vi "Main.vi"(11 "Module Admin":refnum<class "Delacor_lib_QMH_Module Admin.lvclass">) -> ()   [LabVIEW 2023, in "Initial Data.lvlib"]
doc: "This template is based off of the Queued Message Handler design pattern and the Queued Message Handler project template that ships with LabVIEW.\n\nThe main difference is that the queue is private to this module and communication between modules is performed via Broadcast and Request events.\n\nRequest events are wrapped in public API methods and are handled in the Event Handling Loop (EHL) of this VI. Any module can register for Broadcast events sent by this module. The EHL generates messages based on user interface actions.\n\nThe Message Handling Loop (MHL) processes messages generated by the EHL, or by other messages. The messages are string values, so new messages can be added easily to the Message Cases case structure in the MHL. Each message cluster can also provide an optional value for Message Data, which is a variant that can be converted to whatever message-specific data is required.\n_____\nBased on DQMH Project Template 6.1.0.94."
uses:
  Initial Data.lvlib
  <vilib>/Delacor/Delacor QMH/Libraries/Module Admin_class/Delacor_lib_QMH_Module Admin.lvclass
  InitalData Type.ctl
  Module Data--cluster.ctl
  <vilib>/Delacor/Delacor QMH/Libraries/Message Queue_class/Delacor_lib_QMH_Message Queue.lvclass/Delacor_lib_QMH_Message Queue.ctl
  Stop Argument--cluster.ctl
  <vilib>/Delacor/Delacor QMH/Libraries/Module Admin_class/Delacor_lib_QMH_Module Admin.lvclass/Delacor_lib_QMH_Module Admin.ctl
  Update Brod Argument--cluster.ctl
  SubPanel Argument--cluster.ctl
  <vilib>/Utility/miscctls.llb/LVPointTypeDef.ctl
  <vilib>/Delacor/Delacor QMH/Libraries/Message Queue_class/Delacor_lib_QMH_Enqueue Message (Single).vi
  <vilib>/Delacor/Delacor QMH/Libraries/Module Admin_class/Delacor_lib_QMH_Get External Launch.vi
  <vilib>/Utility/error.llb/Error Cluster From Error Code.vi
  <vilib>/ErrorRing/Error Ring.xnode
  <vilib>/Delacor/Delacor QMH/Libraries/Message Queue_class/Delacor_lib_QMH_Message Queue.lvclass
panel:
  in  "Исходные данные":T1
  out "error out":errorcluster
  in  "Simulate MHL Error":bool
  in  "Simulate EHL Error":bool
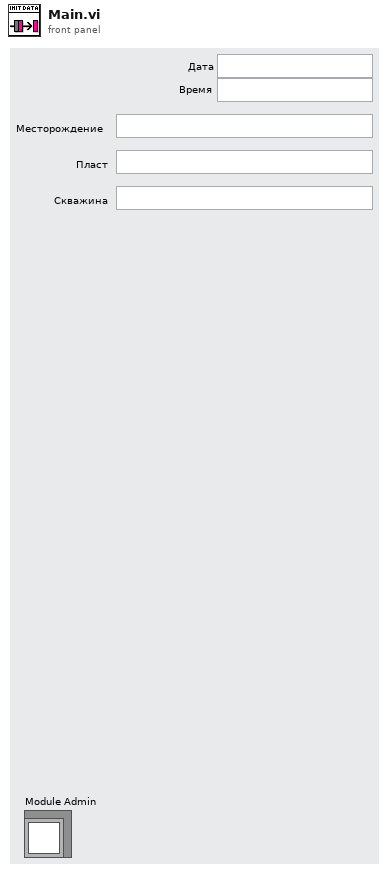
[diagram p1: front panel]
types:
  T1 = typedef "Initial Data.lvlib/InitalData Type.ctl" = cluster{"Дата":string, "Время":string, "Месторождение":string, "Пласт":string, "Скважина":string}
  T2 = typedef "Initial Data.lvlib/Request Events--cluster.ctl" = cluster{"Stop Module":refnum<user-event>, "Show Panel":refnum<user-event>, "Hide Panel":refnum<user-event>, "Get Module Execution Status":refnum<user-event>, "Show Diagram":refnum<user-event>, "Update Brod":refnum<user-event>, "SubPanel":refnum<user-event>}
  T3 = typedef "Initial Data.lvlib/Module Data--cluster.ctl" = cluster{"Status":string, "Исходные данные":T1}
  T4 = enum32{"invalid lock state", "Not Locked", "Locked (No Password)", "Password-protected"}
  T5 = typedef "Initial Data.lvlib/Stop Argument--cluster.ctl" = cluster{"Origin":string, "Exit via Stop Module Req?":bool, "Wait for Module to stop?":bool}
  T6 = typedef "Initial Data.lvlib/Update Brod Argument--cluster.ctl" = cluster{"Boolean":bool}
  T7 = typedef "Initial Data.lvlib/SubPanel Argument--cluster.ctl" = cluster{"Sub Panel":refnum<vi>}
  T8 = typedef "LVPointTypeDef.ctl" = cluster{"Horizontal":i16, "Vertical":i16}
  T9 = enum32{"Invalid", "Standard", "Closed", "Hidden", "Minimized", "Maximized"}
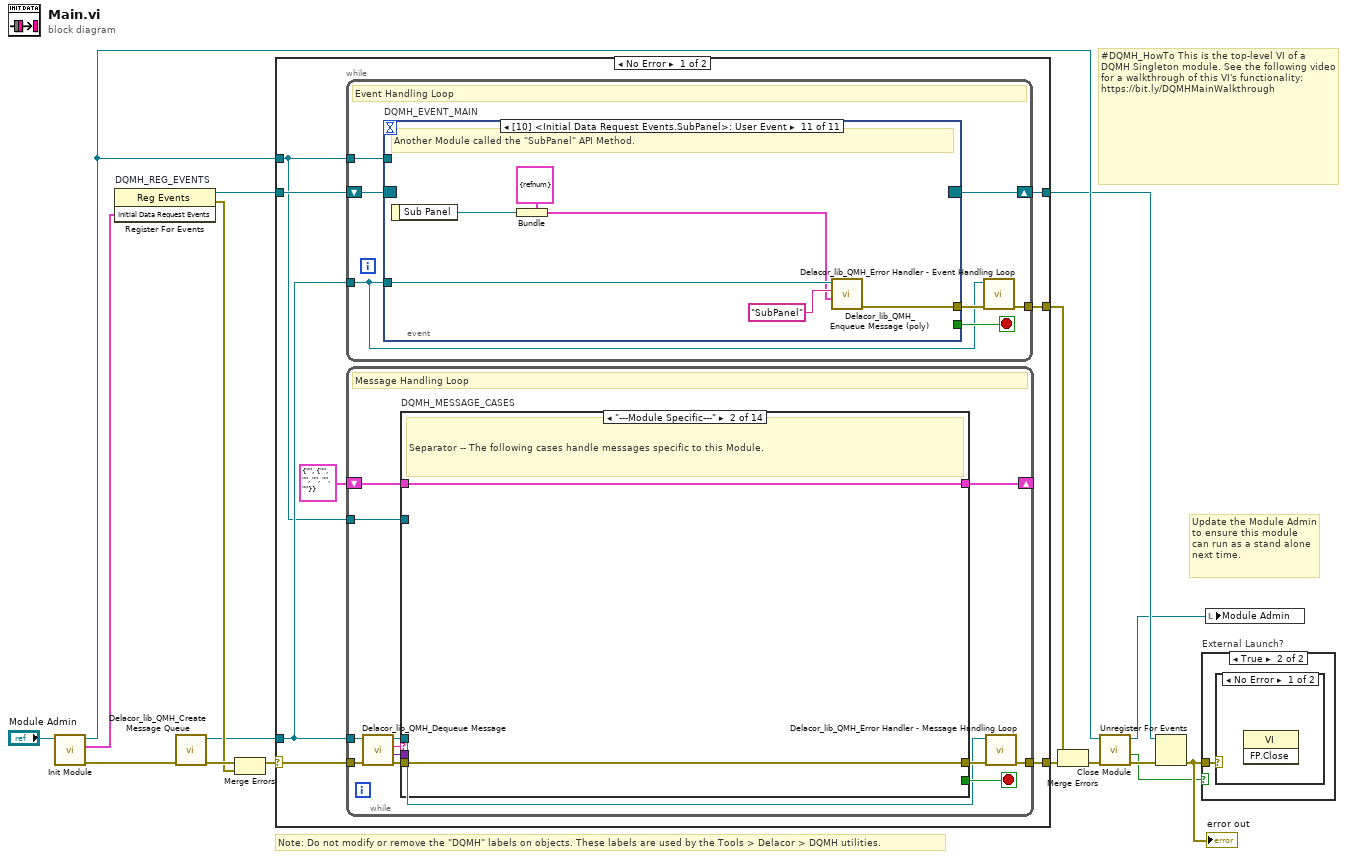
[diagram p0: block diagram]
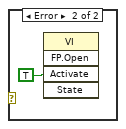
[diagram p3: hidden frame]
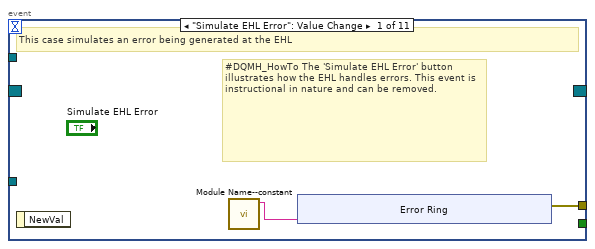
[diagram p4: hidden frame]
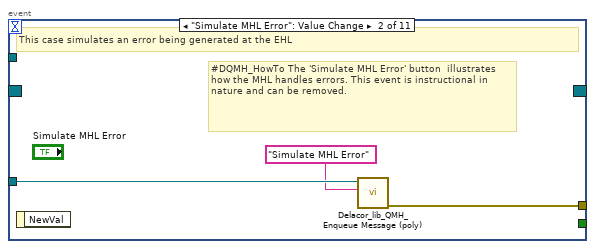
[diagram p5: hidden frame]
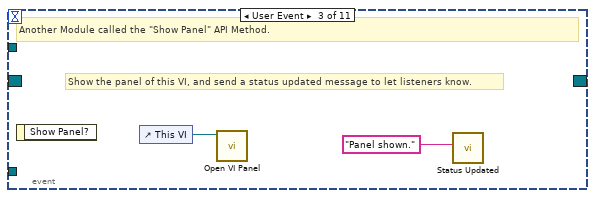
[diagram p6: hidden frame]
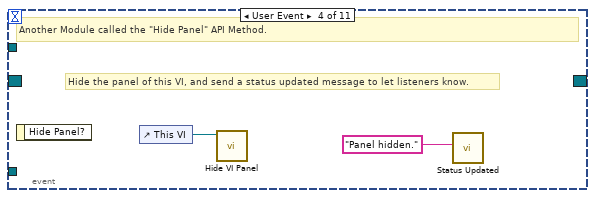
[diagram p7: hidden frame]
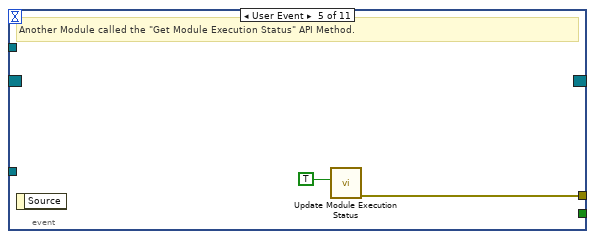
[diagram p8: hidden frame]
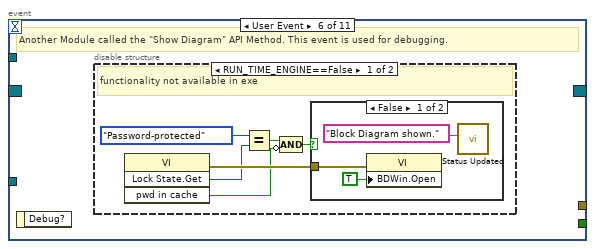
[diagram p9: hidden frame]
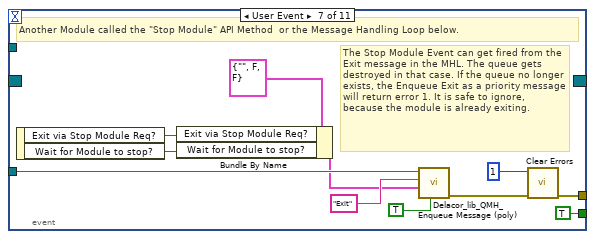
[diagram p12: hidden frame]
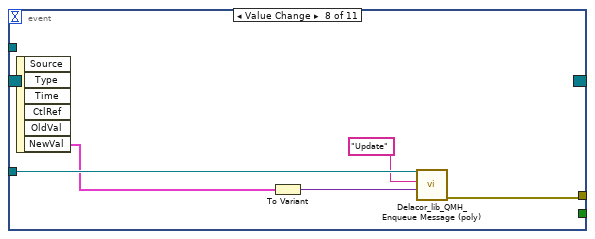
[diagram p13: hidden frame]
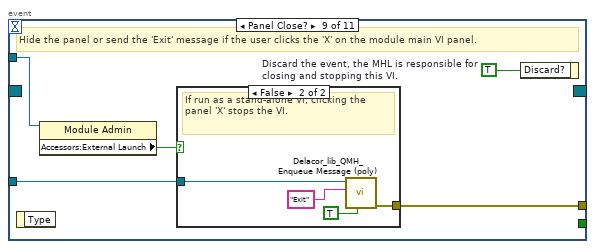
[diagram p14: hidden frame]
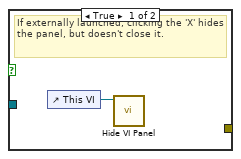
[diagram p15: hidden frame]
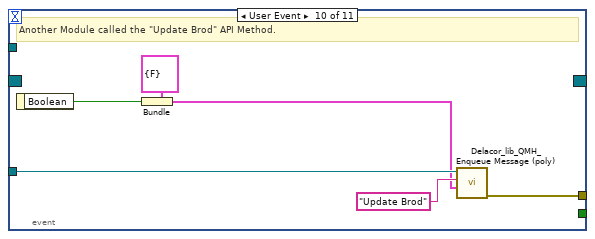
[diagram p16: hidden frame]
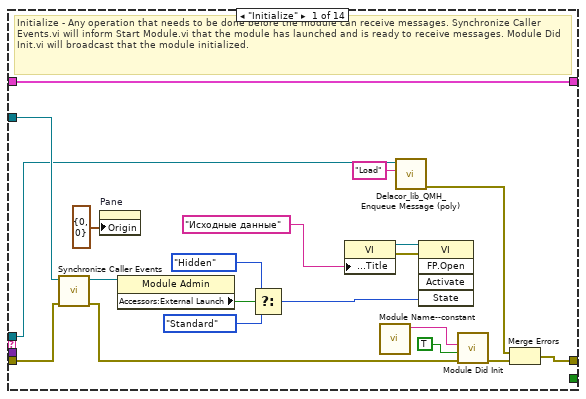
[diagram p17: hidden frame]
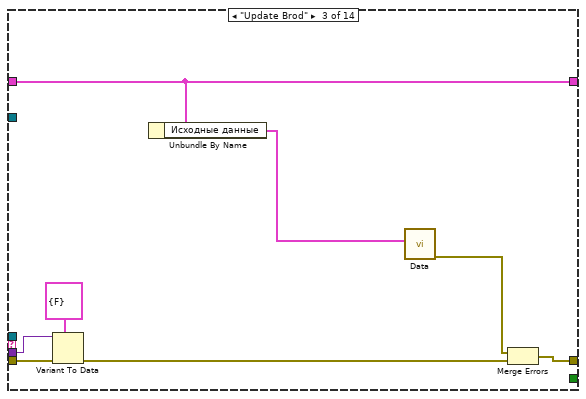
[diagram p18: hidden frame]
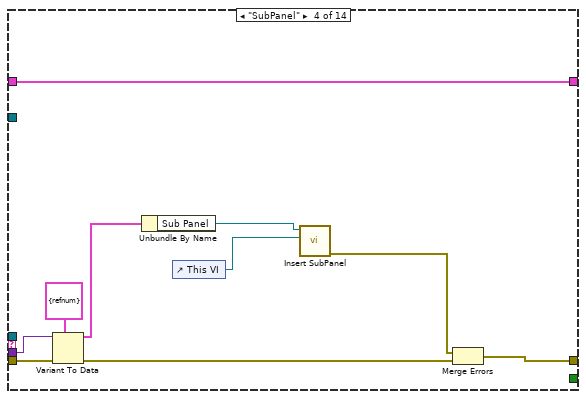
[diagram p19: hidden frame]
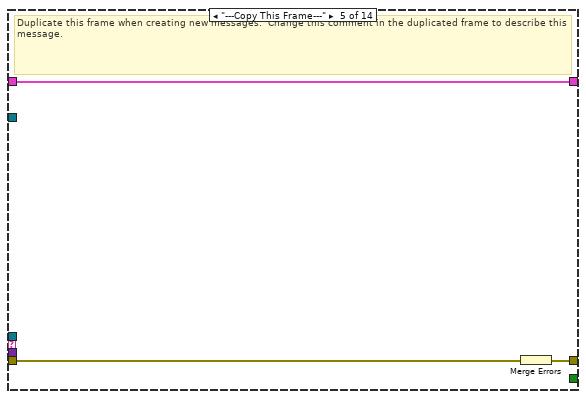
[diagram p20: hidden frame]
diagram:
  # "#DQMH_HowTo This is the top-level VI of a DQMH Singleton module. See the following video for a walkthrough of this VI's functionality: https://bit.ly/DQMHMainWalkthrough"
  # "Note: Do not modify or remove the \"DQMH\" labels on objects. These labels are used by the Tools > Delacor > DQMH utilities."
  # "Update the Module Admin to ensure this module can run as a stand alone next time."
  n1 = call "Init Module.vi"("Singleton Module Admin in"="Module Admin") -> ("error out"=w16:errorcluster, "Initial Data Request Events"=w5:T2, "Singleton Module Admin out"=w8:refnum<class "Delacor_lib_QMH_Module Admin.lvclass">)  [unwired: 8 in]
  n2 = register-events "DQMH_REG_EVENTS"(w5) -> (reference out=w6:refnum<event-registration>, error out=w9:errorcluster)  [unwired: 2 in]
  n3 = call <vilib>:"Delacor_lib_QMH_Create Message Queue.vi"("error in"=w16) -> ("error out"=w11:errorcluster, "Message Queue"=w4:refnum<class "Delacor_lib_QMH_Message Queue.lvclass">)  [unwired: 9 in]
  n4 = Merge Errors(w11, w9) -> (w10:errorcluster)
  n5 = case shown="No Error" w10 {
    selector: w10 -> [w23 w259]
    tunnel: [w25 w258] -> w17
    tunnel: [w22 w264] -> w7
    tunnel: w6 -> [w20 w264]
    tunnel: w4 -> [w19 w257]
    tunnel: [w24 _] -> w14
    tunnel: w8 -> [w18 w260]
    frame No Error {
      n6 = while {
        tunnel: w19 -> [w26]
        shift-right: [w29] -> w22
        shift-left: w20 -> [w30]
        tunnel: [w31] -> w24
        tunnel: w18 -> [w27]
        stop <- w28 stop-if-true
        # "Event Handling Loop"
        n7 = event "DQMH_EVENT_MAIN" shown="[10] <Initial Data Request Events.SubPanel>: User Event" {
          selector: w30 -> [_ _ _ _ _ _ _ _ _ _ _]
          dyn-events: [_ _ _ _ _ _ _ _ _ _ _] -> w29
          timeout: _ -> [_ _ _ _ _ _ _ _ _ _ _]
          tunnel: [_ _ _ _ _ _ TRUE ("Discard?") _ _ _ _] -> w28
          tunnel: w26 -> [_ w43 _ _ _ _ w66 w75 w78 w91 w97]
          tunnel: [w34 w44 _ _ w50 _ w69 w73 w80 w86 w92] -> w32
          tunnel: w27 -> [_ _ _ _ _ _ _ _ w77 _ _]
          event "Simulate EHL Error": Value Change {
            # "#DQMH_HowTo The 'Simulate EHL Error' button  illustrates how the EHL handles errors. This event is instructional in nature and can be removed."
            # "This case simulates an error being generated at the EHL"
            n8 = event-data() -> ()  [unwired: 1 in, 1 out]
            n9 = call "Module Name--constant.vi"() -> ("Module Name"=w33:string)  [unwired: 11 in]
            n10 = xnode "Error Ring"("parameter 0"=w33) -> ("error out"=w34:errorcluster)
          }
          event "Simulate MHL Error": Value Change {
            # "#DQMH_HowTo The 'Simulate MHL Error' button  illustrates how the MHL handles errors. This event is instructional in nature and can be removed."
            # "This case simulates an error being generated at the EHL"
            n11 = event-data() -> ()  [unwired: 1 in, 1 out]
            n12 = call-poly <vilib>:"Delacor_lib_QMH_Enqueue Message (poly).vi"("Message"="Simulate MHL Error", "Message Queue in"=w43) -> ("error out"=w44:errorcluster)  [unwired: 8 in, 1 out]
          }
          event User Event {
            # "Show the panel of this VI, and send a status updated message to let listeners know."
            # "Another Module called the \"Show Panel\" API Method."
            n13 = event-data() -> ()  [unwired: 1 in, 1 out]
            n14 = control-ref of="This VI"() -> (w46:refnum<vi>)
            n15 = call "Open VI Panel.vi"("VI"=w46) -> ()  [unwired: 10 in, 1 out]
            n16 = call "Status Updated.vi"("Status"="Panel shown." ("format string")) -> ()  [unwired: 10 in, 1 out]
          }
          event User Event {
            # "Hide the panel of this VI, and send a status updated message to let listeners know."
            # "Another Module called the \"Hide Panel\" API Method."
            n17 = event-data() -> ()  [unwired: 1 in, 1 out]
            n18 = control-ref of="This VI"() -> (w48:refnum<vi>)
            n19 = call "Hide VI Panel.vi"("VI"=w48) -> ()  [unwired: 10 in, 1 out]
            n20 = call "Status Updated.vi"("Status"="Panel hidden." ("format string")) -> ()  [unwired: 10 in, 1 out]
          }
          event User Event {
            # "Another Module called the \"Get Module Execution Status\" API Method."
            n21 = event-data() -> ()  [unwired: 1 in, 1 out]
            n22 = call "Update Module Execution Status.vi"("Running?"=TRUE) -> ("error out"=w50:errorcluster)  [unwired: 10 in]
          }
          event User Event {
            # "Another Module called the \"Show Diagram\" API Method. This event is used for debugging."
            n23 = event-data() -> ()  [unwired: 1 in, 1 out]
            n24 = disable-structure shown="RUN_TIME_ENGINE==False" {
              frame condition #0 (active) {
                # "functionality not available in exe"
                n25 = invoke class="VI" method="Lock State.Get"() -> (error out=w56:errorcluster, "Get Lock State"=w55:T4, "pwd in cache"=w52:bool)  [unwired: 4 in, 1 out]
                n26 = Equal?(x=T4."Password-protected", y=w55) -> (x = y?=w53:bool)
                n27 = Compound Arithmetic op=AND(w53, invert w52) -> (w51:bool)
                n28 = case shown="False" w51 {
                  tunnel: w56 -> [w59 _]
                  frame False {
                    n29 = property class="VI"(error in=w59, "BDWin.Open"=TRUE ("Block Diagram Window:Open")) -> ()  [unwired: 1 in, 2 out]
                    n30 = call "Status Updated.vi"("Status"="Block Diagram shown." ("format string")) -> ()  [unwired: 10 in, 1 out]
                  }
                  frame True {
                    # "Password-protected VI, and the password is not in the cache. Do not show the diagram."
                  }
                }
              }
              frame condition #1 {
              }
            }
          }
          event User Event {
            # "The Stop Module Event can get fired from the Exit message in the MHL. The queue gets destroyed in that case. If the queue no longer exists, the Enqueue Exit as a priority message will return error 1. It is safe to ignore, because the module is already exiting."
            # "Another Module called the \"Stop Module\" API Method  or the Message Handling Loop below."
            n31 = event-data() -> ("Exit via Stop Module Req?"=w62:bool, "Wait for Module to stop?"=w61:bool)  [unwired: 1 in]
            n32 = Bundle By Name(cluster=T5 {"Origin"="", "Exit via Stop Module Req?"=FALSE, "Wait for Module to stop?"=FALSE} ("Stop Argument"), "Exit via Stop Module Req?"=w62, "Wait for Module to stop?"=w61) -> (w60:T5)
            n33 = call-poly <vilib>:"Delacor_lib_QMH_Enqueue Message (poly).vi"("Priority Message? (F)"=TRUE, "Message Data"=w60, "Message"="Exit", "Message Queue in"=w66) -> ("error out"=w70:errorcluster)  [unwired: 6 in, 1 out]
            n34 = call <vilib>:"Clear Errors.vi"("error in (no error)"=w70, "specific error code to clear (0: all)"=1) -> ("error out"=w69:errorcluster)  [unwired: 4 in, 1 out]
          }
          event Value Change {
            n35 = event-data() -> ("NewVal"=w72:T1)  [unwired: 1 in, 5 out]
            n36 = To Variant(anything=w72) -> (Variant=w71:variant)
            n37 = call-poly <vilib>:"Delacor_lib_QMH_Enqueue Message (poly).vi"("Message Data"=w71, "Message"="Update", "Message Queue in"=w75) -> ("error out"=w73:errorcluster)  [unwired: 7 in, 1 out]
          }
          event Panel Close? {
            w79 = TRUE  # Discard the event, the MHL is responsible for closing and stopping this VI.
            # "Hide the panel or send the 'Exit' message if the user clicks the 'X' on the module main VI panel."
            n38 = event-data() -> ()  [unwired: 1 in, 1 out]
            n39 = property class="Module Admin"(reference=w77) -> ("Accessors:External Launch"=w76:bool)  [unwired: 1 in, 2 out]
            n40 = case shown="False" w76 {
              tunnel: w78 -> [_ w84]
              tunnel: [_ w85] -> w80
              frame True {
                # "If externally launched, clicking the 'X' hides the panel, but doesn't close it."
                n41 = control-ref of="This VI"() -> (w81:refnum<vi>)
                n42 = call "Hide VI Panel.vi"("VI"=w81) -> ()  [unwired: 10 in, 1 out]
              }
              frame False {
                # "If run as a stand-alone VI, clicking the panel 'X' stops the VI."
                n43 = call-poly <vilib>:"Delacor_lib_QMH_Enqueue Message (poly).vi"("Priority Message? (F)"=TRUE, "Message"="Exit", "Message Queue in"=w84) -> ("error out"=w85:errorcluster)  [unwired: 7 in, 1 out]
              }
            }
            n44 = event-data("Discard?"=w79) -> ()  [unwired: 1 in, 1 out]
          }
          event User Event {
            # "Another Module called the \"Update Brod\" API Method."
            n45 = event-data() -> ("Boolean"=w87:bool)  [unwired: 1 in]
            n46 = Bundle(cluster=T6 {"Boolean"=FALSE} ("Update Brod Argument"), "Boolean"=w87) -> (w88:T6)
            n47 = call-poly <vilib>:"Delacor_lib_QMH_Enqueue Message (poly).vi"("Message Data"=w88, "Message"="Update Brod", "Message Queue in"=w91) -> ("error out"=w86:errorcluster)  [unwired: 7 in, 1 out]
          }
          event User Event {
            # "Another Module called the \"SubPanel\" API Method."
            n48 = event-data() -> ("Sub Panel"=w93:refnum<vi>)  [unwired: 1 in]
            n49 = Bundle(cluster=T7 {"Sub Panel"=refnum} ("SubPanel Argument"), "Sub Panel"=w93) -> (w94:T7)
            n50 = call-poly <vilib>:"Delacor_lib_QMH_Enqueue Message (poly).vi"("Message Data"=w94, "Message"="SubPanel", "Message Queue in"=w97) -> ("error out"=w92:errorcluster)  [unwired: 7 in, 1 out]
          }
        }
        n51 = call-dynamic "Delacor_lib_QMH_Error Handler - Event Handling Loop.vi"("error in"=w32, "Message Queue in"=w26) -> ("dup error in"=w31:errorcluster)  [unwired: 8 in, 1 out]
      }
      n52 = while {
        tunnel: w19 -> [w100]
        shift-right: [w104] -> _
        shift-left: T3 {"Status"="", "Исходные данные"={"Дата"="", "Время"="", "Месторождение"="", "Пласт"="", "Скважина"=""}} ("Data Cluster") -> [w105]
        tunnel: w23 -> [w108]
        tunnel: [w106] -> w25
        tunnel: w18 -> [w98]
        stop <- w103 stop-if-true
        # "Message Handling Loop"
        n53 = call-dynamic "Delacor_lib_QMH_Dequeue Message.vi"("error in"=w108, "Message Queue in"=w100) -> ("error out"=w107:errorcluster, "Message Data"=w101:variant, "Message"=w102:string, "Message Queue out"=w99:refnum<class "Delacor_lib_QMH_Message Queue.lvclass">)  [unwired: 6 in]
        n54 = case "DQMH_MESSAGE_CASES" shown="\"---Module Specific---\"" w102 {
          selector: w102 -> [_ _ _ _ _ _ _ _ _ _ _ _ _ w244]
          tunnel: w99 -> [w111 _ _ _ _ w154 w168 w182 _ _ _ w210 w234 _]
          tunnel: w107 -> [w128 w131 w139 w149 w152 w161 w176 w187 w193 w195 w200 w217 w240 w246]
          tunnel: [w113 w131 w135 w143 w151 w160 w175 w186 w192 w195 w199 w213 w237 w247] -> w109
          tunnel: w105 -> [w115 w130 w133 w148 w150 w159 w167 w181 w190 w194 w197 w212 w225 w245]
          tunnel: [w115 w130 w133 w148 w150 w159 w172 w185 w189 w194 w197 w212 w225 w245] -> w104
          tunnel: [_ _ _ _ _ _ _ _ _ _ _ _ w233 _] -> w103
          tunnel: w101 -> [_ _ w137 w146 _ _ w174 _ _ _ _ w211 w232 _]
          tunnel: w98 -> [w120 _ _ _ _ _ _ _ _ _ _ w209 w227 _]
          frame "Initialize" {
            # "Initialize - Any operation that needs to be done before the module can receive messages. Synchronize Caller Events.vi will inform Start Module.vi that the module has launched and is ready to receive messages. Module Did Init.vi will broadcast that the module initialized."
            n55 = call "Synchronize Caller Events.vi"("error in (no error)"=w128, "Singleton Module Admin in"=w120) -> ("error out"=w127:errorcluster, "Singleton Module Admin out"=w117:refnum<class "Delacor_lib_QMH_Module Admin.lvclass">)  [unwired: 8 in]
            n56 = property on="Pane" class="Pane"("Origin"=T8 {"Horizontal"=0, "Vertical"=0}) -> ()  [unwired: 2 in, 2 out]
            n57 = property class="Module Admin"(reference=w117) -> ("Accessors:External Launch"=w124:bool)  [unwired: 1 in, 2 out]
            n58 = Select(t=T9."Hidden" ("State"), s=w124, f=T9."Standard" ("State")) -> (s? t:f=w121:T9)
            n59 = property class="VI"("Front Panel.Title"="Исходные данные" ("Front Panel Window:Title")) -> (reference out=w125:refnum<vi>, error out=w129:errorcluster)  [unwired: 2 in]
            n60 = call "Module Name--constant.vi"() -> ("Module Name"=w118:string)  [unwired: 11 in]
            n61 = call-poly <vilib>:"Delacor_lib_QMH_Enqueue Message (poly).vi"("Message"="Load", "Message Queue in"=w111) -> ("error out"=w112:errorcluster)  [unwired: 8 in, 1 out]
            n62 = invoke class="VI" method="FP.Open"(reference=w125, error in=w129, "State"=w121) -> ()  [unwired: 2 in, 5 out]
            n63 = call "Module Did Init.vi"("error in (no error)"=w127, "Initialized?"=TRUE, "Origin"=w118) -> ("error out"=w126:errorcluster)  [unwired: 8 in]
            n64 = Merge Errors(w112, w126) -> (w113:errorcluster)
          }
          frame "---Module Specific---" {
            # "Separator -- The following cases handle messages specific to this Module."
          }
          frame "Update Brod" {
            n65 = Variant To Data(error in=w139, type=T6 {"Boolean"=FALSE} ("Update Brod Argument"), Variant=w137) -> (error out=w138:errorcluster)  [unwired: 1 out]
            n66 = Unbundle By Name(w133) -> ("Исходные данные"=w132:T1)
            n67 = call "Data.vi"("Исходные данные"=w132) -> ("error out"=w134:errorcluster)  [unwired: 10 in]
            n68 = Merge Errors(w134, w138) -> (w135:errorcluster)
          }
          frame "SubPanel" {
            n69 = Variant To Data(error in=w149, type=T7 {"Sub Panel"=refnum} ("SubPanel Argument"), Variant=w146) -> (data=w144:T7, error out=w147:errorcluster)
            n70 = Unbundle By Name(w144) -> ("Sub Panel"=w141:refnum<vi>)
            n71 = control-ref of="This VI"() -> (w140:refnum<vi>)
            n72 = call "Insert SubPanel.vi"("VI Ref"=w140, "Subpanel Ref"=w141) -> ("error out"=w142:errorcluster)  [unwired: 9 in]
            n73 = Merge Errors(w142, w147) -> (w143:errorcluster)
          }
          frame "---Copy This Frame---" {
            # "Duplicate this frame when creating new messages.  Change this comment in the duplicated frame to describe this message."
            n74 = Merge Errors(w152) -> (w151:errorcluster)
          }
          frame "Load" {
            # "!!!!!!!!!"
            # "Duplicate this frame when creating new messages.  Change this comment in the duplicated frame to describe this message."
            n75 = disable-structure shown="Disabled" {
              disable-tunnel: [w163 _] -> w156
              disable-tunnel: [w162 _] -> w153
              frame Disabled {
                n76 = call "GetFileCFG.vi"() -> ("error out"=w162:errorcluster, "Data"=w163:T1)  [unwired: 2 in]
              }
              frame Enabled {
              }
            }
            n77 = To Variant(anything=w156) -> (Variant=w157:variant)
            n78 = call-poly <vilib>:"Delacor_lib_QMH_Enqueue Message (poly).vi"("Message Data"=w157, "Message"="Update", "Message Queue in"=w154) -> ("error out"=w155:errorcluster)  [unwired: 7 in, 1 out]
            n79 = Merge Errors(w153, w155, w161) -> (w160:errorcluster)
          }
          frame "Update" {
            # "Duplicate this frame when creating new messages.  Change this comment in the duplicated frame to describe this message."
            n80 = Variant To Data(type="Исходные данные", Variant=w174) -> (data=w164:T1, error out=w169:errorcluster)  [unwired: 1 in]
            n81 = Get Date/Time String() -> (date string=w166:string, time string=w165:string)  [unwired: 3 in]
            n82 = Bundle By Name(cluster=w167, "Исходные данные"=w164, "Исходные данные.Дата"=w166, "Исходные данные.Время"=w165) -> (w172:T3)
            n83 = call-poly <vilib>:"Delacor_lib_QMH_Enqueue Message (poly).vi"("Message"="Calculate S", "Message Queue in"=w168) -> ("error out"=w170:errorcluster)  [unwired: 8 in, 1 out]
            n84 = Merge Errors(w170, w169, w176) -> (w175:errorcluster)
          }
          frame "Update data" {
            # "Duplicate this frame when creating new messages.  Change this comment in the duplicated frame to describe this message."
            n85 = Unbundle By Name(w181) -> ("Исходные данные"=w180:T1)
            n86 = Get Date/Time String() -> (date string=w179:string, time string=w178:string)  [unwired: 3 in]
            n87 = Bundle By Name(cluster=w180, "Дата"=w179, "Время"=w178) -> (w177:T1)
            n88 = Bundle By Name(cluster=w181, "Исходные данные"=w177) -> (w185:T3)
            n89 = call-poly <vilib>:"Delacor_lib_QMH_Enqueue Message (poly).vi"("Message"="Calculate S", "Message Queue in"=w182) -> ("error out"=w183:errorcluster)  [unwired: 8 in, 1 out]
            n90 = Merge Errors(w183, w187) -> (w186:errorcluster)
          }
          frame "Calculate S" {
            # "Duplicate this frame when creating new messages.  Change this comment in the duplicated frame to describe this message."
            n91 = Unbundle By Name(w190) -> ("Исходные данные"=w188:T1)
            n92 = local write "Исходные данные"(w188) -> ()
            n93 = Bundle By Name(cluster=w190, "Исходные данные"=w188) -> (w189:T3)
            n94 = call "Data.vi"("Исходные данные"=w188) -> ("error out"=w191:errorcluster)  [unwired: 10 in]
            n95 = Merge Errors(w191, w193) -> (w192:errorcluster)
          }
          frame "---Exit and Error Handling---" {
            # "Separator - The following cases handle errors and exit messages."
          }
          frame "Simulate MHL Error" {
            # "#DQMH_HowTo The 'Simulate MHL Error' button  illustrates how the MHL handles errors. This event is instructional in nature and can be removed."
            # "Simulate an error occurring at the MHL"
            n96 = call "Module Name--constant.vi"() -> ("Module Name"=w196:string)  [unwired: 11 in]
            n97 = xnode "Error Ring"("parameter 0"=w196) -> ("error out"=w198:errorcluster)
            n98 = Merge Errors(w200, w198) -> (w199:errorcluster)
          }
          frame "Error" {
            # "#CodeRecommended - If you ever change the name of this \"Error\" message, you'll need to update the name in the Check Loop Error.vi as well."
            # "#CodeRecommended - If the module is running in standalone mode (External Launch = FALSE), this code will pop up an error dialog and call the 'Exit' message if an error occurs. Add more fine-grained error handling here."
            # "Error - Check the error message data and respond accordingly. This message is sent by the \"Error Handler\" VIs at the end of each loop in this application."
            n99 = property class="Module Admin"(reference=w209) -> ("Accessors:External Launch"=w208:bool)  [unwired: 1 in, 2 out]
            n100 = Variant To Data(error in=w217, type=errorcluster {"status"=FALSE, "code"=0, "source"=""} ("error constant"), Variant=w211) -> (data=w218:errorcluster, error out=w215:errorcluster)
            n101 = call "Error Reported.vi"("Error"=w218) -> ()  [unwired: 10 in, 1 out]
            n102 = case shown="False" w208 {
              tunnel: [w223 _] -> w214
              tunnel: w210 -> [w221 _]
              tunnel: w218 -> [w222 _]
              frame False {
                # "If the module is running standalone, then pop up an error dialog and call the \"Exit\" message."
                n103 = call <vilib>:"Simple Error Handler.vi"("error in (no error)"=w222) -> ()  [unwired: 4 in, 5 out]
                n104 = call-poly <vilib>:"Delacor_lib_QMH_Enqueue Message (poly).vi"("Priority Message? (F)"=TRUE, "Message"="Exit", "Message Queue in"=w221) -> ("error out"=w223:errorcluster)  [unwired: 7 in, 1 out]
              }
              frame True {
                # "If the module was launched externally, calling the Error Reported broadcast VI is the only action performed by the \"Error\" message. The module's caller can then process the error appropriately."
              }
            }
            n105 = Merge Errors(w215, w214) -> (w213:errorcluster)
            n106 = local write "error out"(w213) -> ()
          }
          frame "Exit" {
            w231 = 91  # 91: not all Exit messages will have an argument
            w233 = TRUE  # Stop the VI
            # "!!!!!!!!!"
            # "Release the message queue reference"
            # "Exit - Exit the application."
            n107 = Variant To Data(error in=w240, type=T5 {"Origin"="", "Exit via Stop Module Req?"=FALSE, "Wait for Module to stop?"=FALSE} ("Stop Argument"), Variant=w232) -> (data=w229:T5, error out=w236:errorcluster)
            n108 = Unbundle By Name(w225) -> ("Исходные данные"=w224:T1)
            n109 = call <vilib>:"Clear Errors.vi"("error in (no error)"=w236, "specific error code to clear (0: all)"=w231) -> ("error out"=w239:errorcluster)  [unwired: 4 in, 1 out]
            n110 = control-ref of="This VI"() -> (w228:refnum<vi>)
            n111 = disable-structure shown="Disabled" {
              disable-tunnel: [w242 _] -> w226
              disable-tunnel: w224 -> [w241 _]
              frame Disabled {
                n112 = call "SaveFileCFG.vi"("Data"=w241) -> ("error out"=w242:errorcluster)  [unwired: 2 in]
              }
              frame Enabled {
              }
            }
            n113 = call-dynamic "Delacor_lib_QMH_Release Message Queue.vi"("error in"=w239, "Message Queue"=w234) -> ("error out"=w238:errorcluster)  [unwired: 9 in]
            n114 = call "Handle Exit.vi"("Stop Argument"=w229, "Admin in"=w227, "VI reference"=w228) -> ("error out"=w235:errorcluster)  [unwired: 7 in, 1 out]
            n115 = Merge Errors(w226, w238, w235) -> (w237:errorcluster)
          }
          frame Default {
            # "'Default' case only runs if there is a message that isn't defined in any of the other cases.  Output a programming error."
            n116 = call "Module Name--constant.vi"() -> ("Module Name"=w243:string)  [unwired: 11 in]
            n117 = xnode "Error Ring"("parameter 0"=w244, "parameter 1"=w243) -> ("error out"=w248:errorcluster)
            n118 = Merge Errors(w246, w248) -> (w247:errorcluster)
          }
        }
        n119 = call-dynamic "Delacor_lib_QMH_Error Handler - Message Handling Loop.vi"("error in"=w109, "Message Queue in"=w99) -> ("dup error in"=w106:errorcluster)  [unwired: 8 in, 1 out]
      }
    }
    frame Error {
      # "Synchronize Caller Events.vi will inform Start Module.vi that the module has launched and will let the code calling Start Module.vi register for broadcasts and would permit the caller receive the broadcast that an error occurred at launch time."
      n120 = call-dynamic "Delacor_lib_QMH_Release Message Queue.vi"("error in"=w259, "Message Queue"=w257) -> ("error out"=w258:errorcluster)  [unwired: 9 in]
      n121 = call "Synchronize Caller Events.vi"("Singleton Module Admin in"=w260) -> ("error out"=w265:errorcluster)  [unwired: 9 in, 1 out]
      n122 = call "Module Name--constant.vi"() -> ("Module Name"=w263:string)  [unwired: 11 in]
      n123 = Format Into String(format string="An error occurred during initialization. %s is no longer running.", w263) -> (resulting string=w261:string)  [unwired: 2 in, 1 out]
      n124 = Merge Errors(w258, w265) -> (w266:errorcluster)
      n125 = call "Error Reported.vi"("Additional Information"=w261, "Error"=w266) -> ()  [unwired: 9 in, 1 out]
    }
  }
  n126 = Merge Errors(w14, w17) -> (w13:errorcluster)
  n127 = call "Close Module.vi"("error in (no error)"=w13, "Module Admin in"=w8) -> ("error out"=w15:errorcluster, "External Launch"=w1:bool, "Module Admin out"=w2:refnum<class "Delacor_lib_QMH_Module Admin.lvclass">)  [unwired: 7 in]
  n128 = Unregister For Events(event registration refnum=w7, error in=w15) -> (error out=w12:errorcluster)
  "error out" <- w12
  n129 = case "External Launch?" shown="True" w1 {
    tunnel: w12 -> [_ w267]
    frame False {
    }
    frame True {
      n130 = case shown="No Error" w267 {
        frame No Error {
          n131 = invoke class="VI" method="FP.Close"() -> ()  [unwired: 3 in, 3 out]
        }
        frame Error {
          n132 = invoke class="VI" method="FP.Open"("Activate"=TRUE ("Activate?")) -> ()  [unwired: 4 in, 5 out]
        }
      }
    }
  }
  n133 = local write "Module Admin"(w2) -> ()
